vi "testCQTDDS.vi"() -> ()   [LabVIEW 2009]
uses:
  C:/Program Files/National Instruments/LabVIEW 2009/instr.lib/CQT_DDS/DDSLibrary/20111108/CQTAD9958.dll
panel:
  in  "Array":dbl[](array[numeric])
  in  "masterReset":bool
  in  "Amplitude (max 1023=1Vpp)":i32=1023
  out "SerialNumber":string
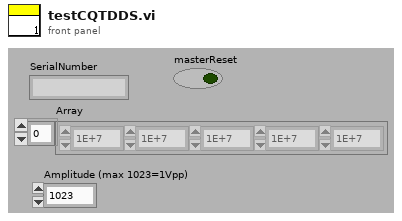
[diagram p1: front panel]
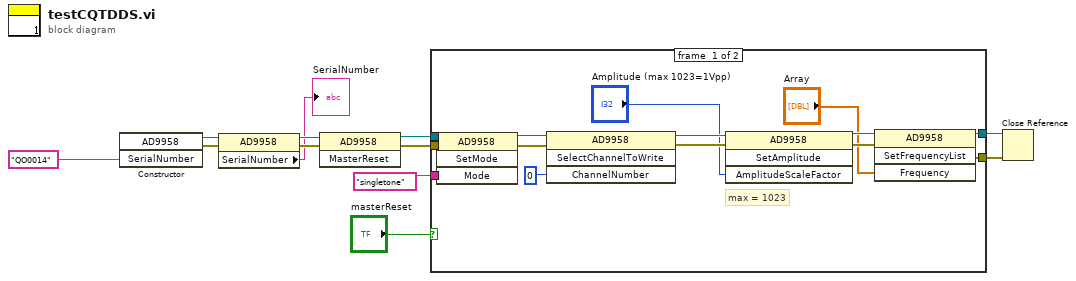
[diagram p0: block diagram]
diagram:
  n1 = constructor class="AD9958"("SerialNumber"="QO0014") -> (reference out=w1:refnum<k24>, error out=w3:errorcluster)  [unwired: 3 in, 2 out]
  n2 = property class="AD9958"(reference=w1, error in=w3) -> (reference out=w7:refnum<k24>, error out=w6:errorcluster, "SerialNumber"=→"SerialNumber":string)
  n3 = invoke class="AD9958" method="MasterReset"(reference=w7, error in=w6) -> (reference out=w12:refnum<k24>, error out=w11:errorcluster)  [unwired: 1 in, 1 out]
  n4 = case shown="False" "masterReset" {
    tunnel: w12 -> [w26 w28]
    tunnel: w11 -> [w25 w27]
    tunnel: "singletone" -> [w24 _]
    tunnel: [w23 w28] -> w9
    tunnel: [w22 w27] -> w8
    frame #0 {
      # "max = 1023"
      n5 = invoke class="AD9958" method="SetMode"(reference=w26, error in=w25, "Mode"=w24) -> (reference out=w15:refnum<k24>, error out=w14:errorcluster)  [unwired: 1 in, 2 out]
      n6 = invoke class="AD9958" method="SelectChannelToWrite"(reference=w15, error in=w14, "ChannelNumber"=0) -> (reference out=w20:refnum<k24>, error out=w19:errorcluster)  [unwired: 1 in, 2 out]
      n7 = invoke class="AD9958" method="SetAmplitude"(reference=w20, error in=w19, "AmplitudeScaleFactor"="Amplitude (max 1023=1Vpp)") -> (reference out=w17:refnum<k24>, error out=w16:errorcluster)  [unwired: 1 in, 2 out]
      n8 = invoke class="AD9958" method="SetFrequencyList"(reference=w17, error in=w16, "Frequency"="Array") -> (reference out=w23:refnum<k24>, error out=w22:errorcluster)  [unwired: 1 in, 2 out]
    }
    frame #1 {
    }
  }
  n9 = Close Reference(reference=w9, error in (no error)=w8) -> ()  [unwired: 1 out]
